vi "InitDeviceManager.vi"(8 "error in (no error)":errorcluster, 9 "start ICL on local host?":bool, 10 "WS Server Port":string="25010", 11 "WS Server IP":string="ws://127.0.0.1") -> (0 "error out":errorcluster, 3 "device manager":refnum<class "DeviceManager.lvclass">)   [LabVIEW 2023, in "DeviceManager.lvclass"]
uses:
  DeviceManager.lvclass
  DeviceManager.lvclass/DeviceManager.ctl
  32339246-19d0-4101-aa43-29dff1db1305.vi
  Source/Classes/Communicator/Communicator.lvclass
panel:
  # "Connector Pane"
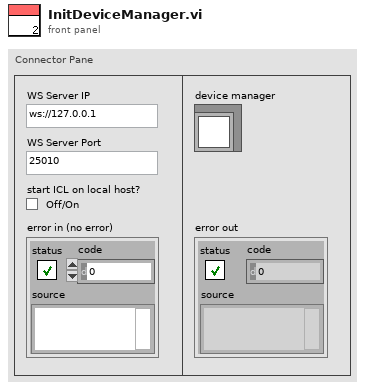
[diagram p1: front panel]
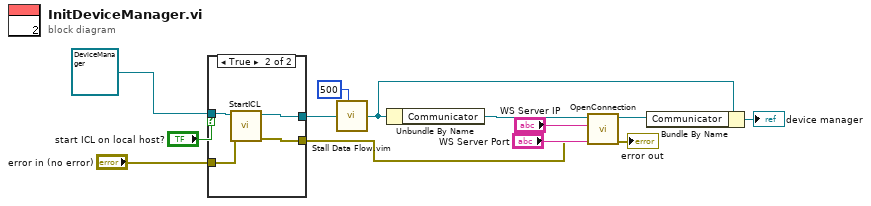
[diagram p0: block diagram]
diagram:
  n1 = case shown="True" "start ICL on local host?" {
    tunnel: refnum<class "DeviceManager.lvclass"> refnum ("DeviceManager.lvclass") -> [w15 w19]
    tunnel: [w15 w18] -> w11
    tunnel: "error in (no error)" -> [w14 w17]
    tunnel: [w14 w16] -> w6
    frame False {
    }
    frame True {
      n2 = call-dynamic "StartICL.vi"("error in (no error)"=w17, "DeviceManager in"=w19) -> ("error out"=w16:errorcluster, "DeviceManager out"=w18:refnum<class "DeviceManager.lvclass">)  [unwired: 8 in]
    }
  }
  n3 = call "Stall Data Flow.vim"("value in"=w11, "milliseconds to wait"=u32 500) -> ("value out"=w5:refnum<class "DeviceManager.lvclass">)  [unwired: 1 out]
  n4 = Unbundle By Name(w5) -> ("Communicator"=w10:refnum<class "Communicator.lvclass">)
  n5 = call-dynamic "OpenConnection.vi"("error in (no error)"=w6, "WS Server Port"="WS Server Port", "WS Server IP"="WS Server IP", "Communicator in"=w10) -> ("error out"=→"error out":errorcluster, "Communicator out"=w4:refnum<class "Communicator.lvclass">)  [unwired: 5 in, 1 out]
  n6 = Bundle By Name(cluster=w5, "Communicator"=w4) -> (→"device manager":refnum<class "DeviceManager.lvclass">)
